vi "PrecessFortran.vi"(0 "Asc reta":string="6.014379870", 1 "Var RA":string="0", 5 "Declinação":string="-0.024612536", 7 "Temperatura (Kelvin)":string="286.45", 9 "Pressao atmosferica (mB)":string="1014", 11 "Humidade relativa (0 a 1)":string=".80", 12 "Var DEC":string="0") -> (3 "Estimated air mass":dbl, 4 "Observed RA (radians)":dbl, 6 "Observed Dec (radians)":dbl, 8 "Observed HA (radians)":dbl, 10 "Local apparent sidereal time (radians)":dbl, 14 "Observed Azimuth (radians: N=0,E=90)":dbl, 15 "Observed Zenith Distance (radians)":dbl)   [LabVIEW 2018]
uses:
  Global_Telescopio.vi
panel:
  in  "Case Constant\n(See Context Help)":bool=TRUE
  out "concatenated string":string
  in  "Taxa de lapso troposferico (Kelvin/metro)":string=".0065"
  in  "Comprimento de onda efetivo (micron)":string=".55"
  in  "Altitude do telescopio":string="1836.4"
  in  "Latitude do telescopio":string="-0.393299281"
  in  "Longitude do telescopio":string="-0.795507013"
  in  "Coord. y do mov. do polo":string="0.000002363"
  in  "Coord. x do mov. do polo":string="0.000000206"
  in  "Delta UT: UT1-UTC":string="-.0776422"
  in  "Data Juliana Modificada":string="54302.384"
  in  "Epoca do equinocio":string="2000"
  in  "Paralaxe":string="0"
  in  "Vel Radial km/seg":string="0"
  out "Arquivo input.txt":string
  out "Arquivo Output.txt":string
  # "Variáveis de entrada"
  # "Variáveis internas"
  # "Constantes"
  # "Variáveis de Saídas"
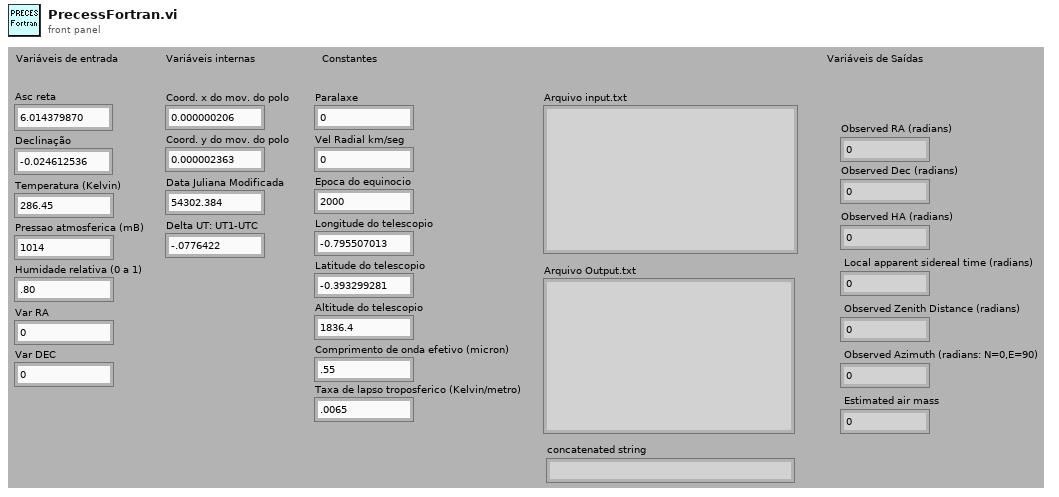
[diagram p1: front panel]
types:
  T1 = enum16{"open", "open or create", "create or replace", "create", "open (read only)"}
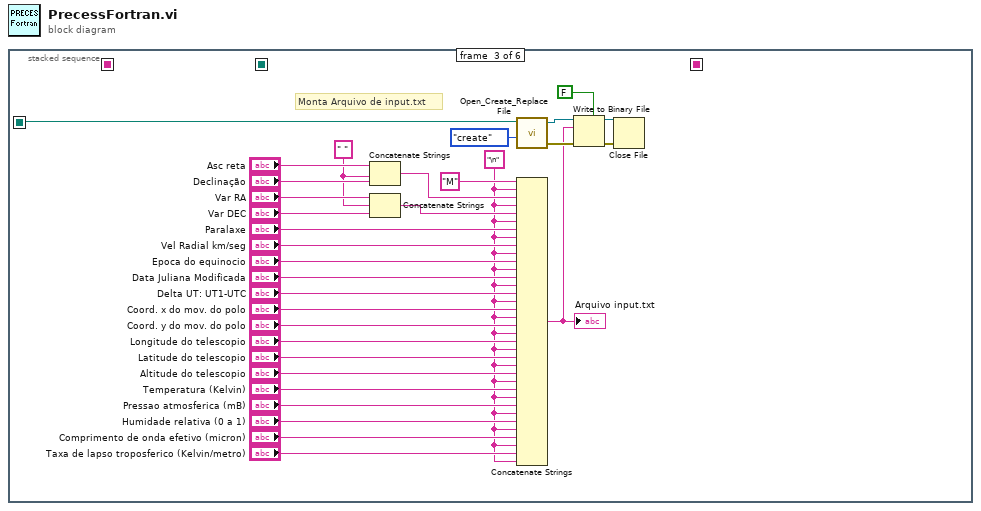
[diagram p0: block diagram]
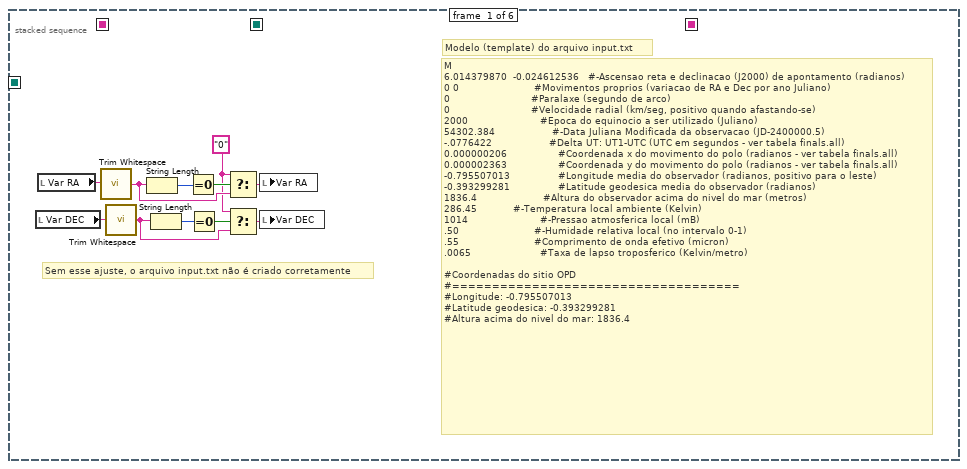
[diagram p2: hidden frame]
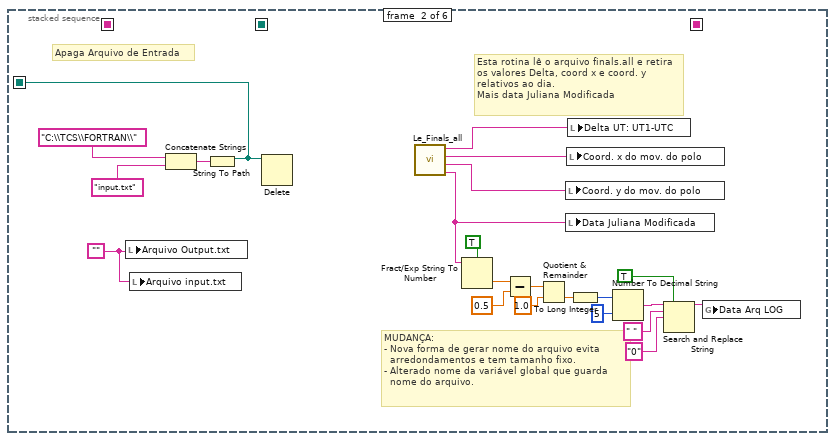
[diagram p3: hidden frame]
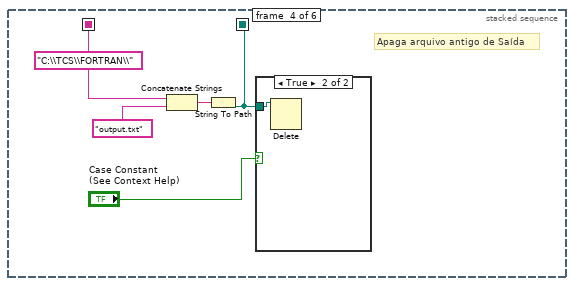
[diagram p4: hidden frame]
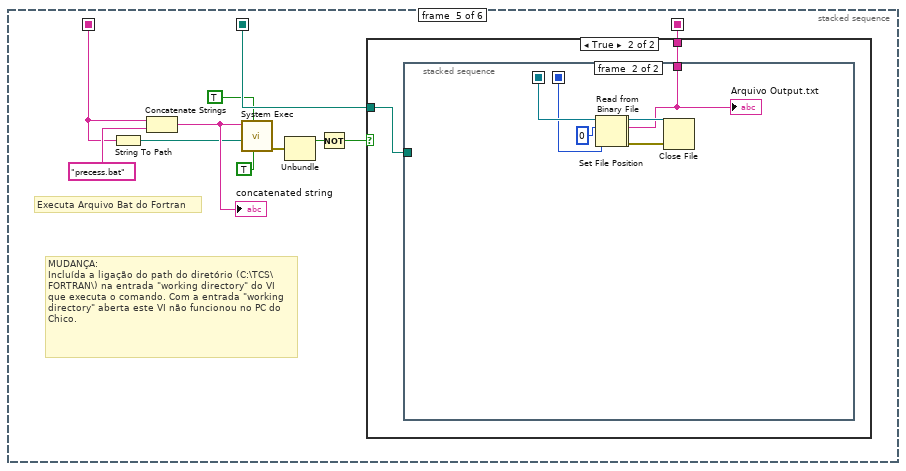
[diagram p6: hidden frame]
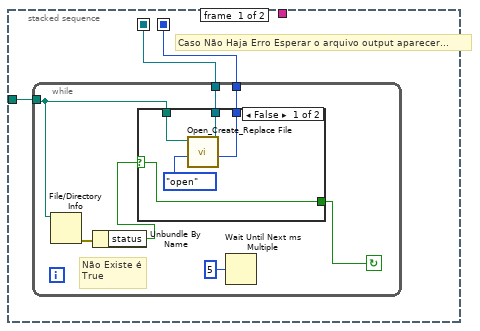
[diagram p8: hidden frame]
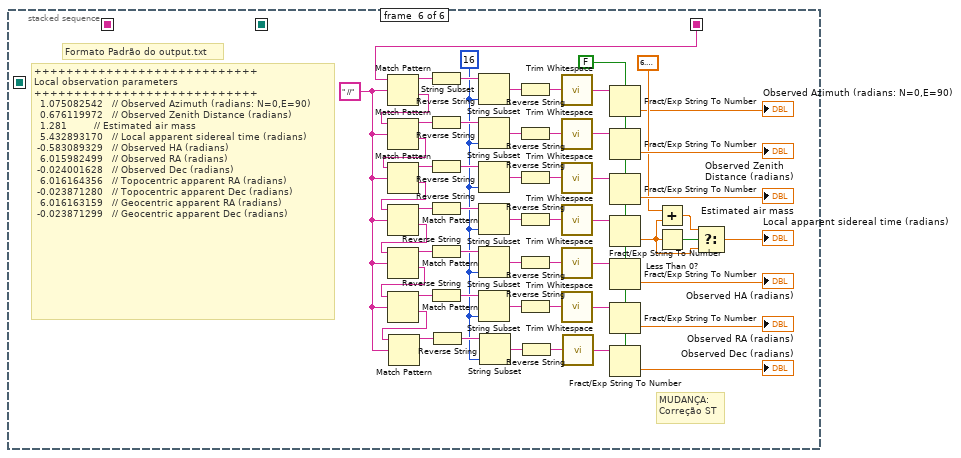
[diagram p10: hidden frame]
diagram:
  n1 = stacked-sequence {
    seq-local: [_ _ _ w70 _ _] -> [_ _ _ _ w72 _]
    seq-local: [_ _ _ w69 _ _] -> [_ _ _ _ w77 _]
    seq-local: [_ w30 _ _ _ _] -> [_ _ w61 _ _ _]
    seq-local: [_ _ _ _ w74 _] -> [_ _ _ _ _ w164]
    frame #0 {
      w3 = "0"
      # "Sem esse ajuste, o arquivo input.txt não é criado corretamente"
      # "Modelo (template) do arquivo input.txt"
      # "M\n6.014379870  -0.024612536   #-Ascensao reta e declinacao (J2000) de apontamento (radianos)\n0 0                         #Movimentos proprios (variacao de RA e Dec por ano Juliano)\n0                           #Paralaxe (segundo de arco)\n0                           #Velocidade radial (km/seg, positivo quando afastando-se)\n2000                        #Epoca do equinocio a ser utilizado (Juliano)\n54302.384                   #-Data Juliana Modificada da observacao (JD-2400000.5)\n-.0776422                   #Delta UT: UT1-UTC (UTC em segundos - ver tabela finals.all)\n0.000000206                 #Coordenada x do movimento do polo (radianos - ver tabela finals.all)\n0.000002363                 #Coordenada y do movimento do polo (radianos - ver tabela finals.all)\n-0.795507013                #Longitude media do observador (radianos, positivo para o leste)\n-0.393299281                #Latitude geodesica media do observador (radianos)\n1836.4                      #Altura do observador acima do nivel do mar (metros)\n286.45      \t\t    #-Temperatura local ambiente (Kelvin)\n1014                        #-Pressao atmosferica local (mB)\n.50                         #-Humidade relativa local (no intervalo 0-1)\n.55                         #Comprimento de onda efetivo (micron)\n.0065                       #Taxa de lapso troposferico (Kelvin/metro)\n\n#Coordenadas do sitio OPD\n#====================================\n#Longitude: -0.795507013\n#Latitude geodesica: -0.393299281\n#Altura acima do nivel do mar: 1836.4"
      n2 = local read "Var DEC"() -> (w10:string)
      n3 = local read "Var RA"() -> (w11:string)
      n4 = call <vilib>:"Trim Whitespace.vi"("string"=w11) -> ("trimmed string"=w5:string)  [unwired: 1 in]
      n5 = call <vilib>:"Trim Whitespace.vi"("string"=w10) -> ("trimmed string"=w4:string)  [unwired: 1 in]
      n6 = String Length(string=w5) -> (length=w9:i32)
      n7 = String Length(string=w4) -> (length=w8:i32)
      n8 = Equal To 0?(x=w9) -> (x = 0?=w7:bool)
      n9 = Equal To 0?(x=w8) -> (x = 0?=w6:bool)
      n10 = Select(t=w3, s=w7, f=w5) -> (s? t:f=w2:string)
      n11 = Select(t=w3, s=w6, f=w4) -> (s? t:f=w1:string)
      n12 = local write "Var RA"(w2) -> ()
      n13 = local write "Var DEC"(w1) -> ()
    }
    frame #1 {
      w29 = ""
      # "MUDANÇA:\n- Nova forma de gerar nome do arquivo evita\n  arredondamentos e tem tamanho fixo.\n- Alterado nome da variável global que guarda\n  nome do arquivo."
      # "Esta rotina lê o arquivo finals.all e retira\nos valores Delta, coord x e coord. y \nrelativos ao dia.\nMais data Juliana Modificada"
      # "Apaga Arquivo de Entrada"
      n14 = local write "Arquivo Output.txt"(w29) -> ()
      n15 = local write "Arquivo input.txt"(w29) -> ()
      n16 = Concatenate Strings("C:\\TCS\\FORTRAN\\", "input.txt") -> (w33:string)
      n17 = String To Path(string=w33) -> (path=w30:path)
      n18 = Delete(path (use dialog)=w30) -> ()  [unwired: 4 in, 3 out]
      n19 = call "Le_Finals_all.vi"() -> ("Data Juliana Modificada"=w25:string, "Saída coord y"=w26:string, "Saída coord x"=w27:string, "Saída DeltaUT"=w28:string)  [unwired: 5 in]
      n20 = Fract/Exp String To Number(use system decimal point (T)=TRUE, string=w25) -> (number=w23:dbl)  [unwired: 2 in, 1 out]
      n21 = Subtract(x=w23, y=0.5) -> (x-y=w13:dbl)
      n22 = Quotient & Remainder(x=w13, y=1.0) -> (floor(x/y)=w15:dbl)  [unwired: 1 out]
      n23 = local write "Coord. y do mov. do polo"(w26) -> ()
      n24 = local write "Data Juliana Modificada"(w25) -> ()
      n25 = local write "Coord. x do mov. do polo"(w27) -> ()
      n26 = local write "Delta UT: UT1-UTC"(w28) -> ()
      n27 = To Long Integer(number=w15) -> (32bit integer=w14:i32)
      n28 = Number To Decimal String(number=w14, width (-)=i16 5) -> (decimal integer string=w20:string)
      n29 = Search and Replace String(replace all?=TRUE ("replace all? (F)"), input string=w20, search string=" ", replace string="0" ("replace string (\"\")")) -> (result string=w12:string)  [unwired: 4 in, 3 out]
      n30 = global write "Global_Telescopio.vi" "Data Arq LOG"(w12) -> ()
    }
    frame #2 {
      w53 = " " ("string")
      w35 = "\n"
      # "Monta Arquivo de input.txt"
      n31 = Concatenate Strings("Asc reta", w53, "Declinação") -> (w57:string)
      n32 = Concatenate Strings("Var RA", w53, "Var DEC") -> (w51:string)
      n33 = call <vilib>:"Open_Create_Replace File.vi"("function (open:0)"=T1."create", "file path"=w61) -> ("error out"=w64:errorcluster, "refnum"=w65:refnum<file>)  [unwired: 6 in, 2 out]
      n34 = Concatenate Strings("M", w35, w57, w35, w51, w35, "Paralaxe", w35, "Vel Radial km/seg", w35, "Epoca do equinocio", w35, "Data Juliana Modificada", w35, "Delta UT: UT1-UTC", w35, "Coord. x do mov. do polo", w35, "Coord. y do mov. do polo", w35, "Longitude do telescopio", w35, "Latitude do telescopio", w35, "Altitude do telescopio", w35, "Temperatura (Kelvin)", w35, "Pressao atmosferica (mB)", w35, "Humidade relativa (0 a 1)", w35, "Comprimento de onda efetivo (micron)", w35, "Taxa de lapso troposferico (Kelvin/metro)", w35) -> (w58:string)
      "Arquivo input.txt" <- w58
      n35 = Write to Binary File(file (use dialog)=w65, data=w58, error in=w64, 5:FALSE ("prepend array or string size? (T)")) -> (refnum out=w62:refnum<file>, error out=w63:errorcluster)  [unwired: 2 in, 1 out]
      n36 = Close File(refnum=w62, error in=w63) -> ()  [unwired: 2 out]
    }
    frame #3 {
      w70 = "C:\\TCS\\FORTRAN\\"
      # "Apaga arquivo antigo de Saída"
      n37 = Concatenate Strings(w70, "output.txt") -> (w68:string)
      n38 = String To Path(string=w68) -> (path=w69:path)
      n39 = case shown="True" "Case Constant\n(See Context Help)" {
        tunnel: w69 -> [_ w71]
        frame False {
        }
        frame True {
          n40 = Delete(path (use dialog)=w71) -> ()  [unwired: 4 in, 3 out]
        }
      }
    }
    frame #4 {
      # "MUDANÇA:\nIncluída a ligação do path do diretório (C:\\TCS\\FORTRAN\\) na entrada \"working directory\" do VI que executa o comando. Com a entrada \"working directory\" aberta este VI não funcionou no PC do Chico."
      # "Executa Arquivo Bat do Fortran"
      n41 = String To Path(string=w72) -> (path=w73:path)
      n42 = Concatenate Strings(w72, "precess.bat") -> (w81:string)
      "concatenated string" <- w81
      n43 = call <vilib>:"System Exec.vi"("run minimized? (F)"=TRUE, "wait until completion? (T)"=TRUE, "working directory"=w73, "command line"=w81) -> ("error out"=w80:errorcluster)  [unwired: 4 in, 3 out]
      n44 = Unbundle(w80) -> ("status"=w79:bool)  [unwired: 2 out]
      n45 = Not(x=w79) -> (.not. x?=w78:bool)
      n46 = case shown="True" w78 {
        tunnel: w77 -> [_ w84]
        tunnel: [_ w83] -> w74
        frame False {
        }
        frame True {
          n47 = stacked-sequence {
            seq-local: [w86 _] -> [_ w108]
            seq-local: [w85 _] -> [_ w104]
            tunnel: w84 -> [w87 _]
            tunnel: [_ w103] -> w83
            frame #0 {
              # "Caso Não Haja Erro Esperar o arquivo output aparecer..."
              n48 = while {
                tunnel: w87 -> [w90]
                tunnel: [w92] -> w86
                tunnel: [w93] -> w85
                stop <- w88 continue-if-true
                # "Não Existe é\nTrue"
                n49 = File/Directory Info(path=w90) -> (error out=w91:errorcluster)  [unwired: 1 in, 6 out]
                n50 = Unbundle By Name(w91) -> ("status"=w89:bool)
                n51 = case shown="False" w89 {
                  selector: w89 -> [w95 w100]
                  tunnel: w90 -> [w99 _]
                  tunnel: [w97 _] -> w93
                  tunnel: [w96 _] -> w92
                  tunnel: [w95 w100] -> w88
                  frame False {
                    n52 = call <vilib>:"Open_Create_Replace File.vi"("function (open:0)"=T1."open", "file path"=w99) -> ("file size (bytes)"=w97:i32, "refnum"=w96:refnum<file>)  [unwired: 6 in, 2 out]
                  }
                  frame True {
                  }
                }
                n53 = Wait Until Next ms Multiple(millisecond multiple=u32 5) -> ()  [unwired: 1 out]
              }
            }
            frame #1 {
              n54 = Set File Position(offset (in bytes) (0)=0 ("pos offset (0)"), refnum=w108) -> (refnum out=w102:refnum<file>, error out=w101:errorcluster)  [unwired: 2 in]
              n55 = Read from Binary File(8:w101, 10:w104, 11:w102) -> (0:w106:errorcluster, 2:w103:string, 3:w107:refnum<file>)  [unwired: 3 in, 1 out]
              "Arquivo Output.txt" <- w103
              n56 = Close File(refnum=w107, error in=w106) -> ()  [unwired: 2 out]
            }
          }
        }
      }
    }
    frame #5 {
      w120 = FALSE ("use system decimal point (T)")
      w129 = 16 ("length (rest)")
      w128 = " //" ("regular expression")
      # "MUDANÇA:\nCorreção ST"
      # "Formato Padrão do output.txt"
      # "++++++++++++++++++++++++++++\nLocal observation parameters\n++++++++++++++++++++++++++++\n  1.075082542   // Observed Azimuth (radians: N=0,E=90) \n  0.676119972   // Observed Zenith Distance (radians) \n  1.281         // Estimated air mass \n  5.432893170   // Local apparent sidereal time (radians) \n -0.583089329   // Observed HA (radians) \n  6.015982499   // Observed RA (radians) \n -0.024001628   // Observed Dec (radians) \n  6.016164356   // Topocentric apparent RA (radians) \n -0.023871280   // Topocentric apparent Dec (radians) \n  6.016163159   // Geocentric apparent RA (radians) \n -0.023871299   // Geocentric apparent Dec (radians)"
      n57 = Match Pattern(string=w164, regular expression=w128) -> (before substring=w163:string, after substring=w151:string)  [unwired: 1 in, 2 out]
      n58 = Match Pattern(string=w151, regular expression=w128) -> (before substring=w156:string, after substring=w150:string)  [unwired: 1 in, 2 out]
      n59 = Match Pattern(string=w150, regular expression=w128) -> (before substring=w155:string, after substring=w133:string)  [unwired: 1 in, 2 out]
      n60 = Match Pattern(string=w133, regular expression=w128) -> (before substring=w149:string, after substring=w132:string)  [unwired: 1 in, 2 out]
      n61 = Match Pattern(string=w132, regular expression=w128) -> (before substring=w145:string, after substring=w131:string)  [unwired: 1 in, 2 out]
      n62 = Match Pattern(string=w131, regular expression=w128) -> (before substring=w141:string, after substring=w130:string)  [unwired: 1 in, 2 out]
      n63 = Match Pattern(string=w130, regular expression=w128) -> (before substring=w134:string)  [unwired: 1 in, 3 out]
      n64 = Reverse String(1:w163) -> (0:w162:string)
      n65 = Reverse String(1:w156) -> (0:w157:string)
      n66 = Reverse String(1:w155) -> (0:w154:string)
      n67 = Reverse String(1:w149) -> (0:w148:string)
      n68 = Reverse String(1:w145) -> (0:w144:string)
      n69 = Reverse String(1:w141) -> (0:w140:string)
      n70 = Reverse String(1:w134) -> (0:w135:string)
      n71 = String Subset(string=w162, length (rest)=w129) -> (substring=w161:string)  [unwired: 1 in]
      n72 = String Subset(string=w157, length (rest)=w129) -> (substring=w158:string)  [unwired: 1 in]
      n73 = String Subset(string=w154, length (rest)=w129) -> (substring=w153:string)  [unwired: 1 in]
      n74 = String Subset(string=w148, length (rest)=w129) -> (substring=w147:string)  [unwired: 1 in]
      n75 = String Subset(string=w144, length (rest)=w129) -> (substring=w143:string)  [unwired: 1 in]
      n76 = String Subset(string=w140, length (rest)=w129) -> (substring=w139:string)  [unwired: 1 in]
      n77 = String Subset(string=w135, length (rest)=w129) -> (substring=w136:string)  [unwired: 1 in]
      n78 = Reverse String(1:w161) -> (0:w160:string)
      n79 = Reverse String(1:w158) -> (0:w159:string)
      n80 = Reverse String(1:w153) -> (0:w152:string)
      n81 = Reverse String(1:w147) -> (0:w146:string)
      n82 = Reverse String(1:w143) -> (0:w142:string)
      n83 = Reverse String(1:w139) -> (0:w138:string)
      n84 = Reverse String(1:w136) -> (0:w137:string)
      n85 = call <vilib>:"Trim Whitespace.vi"("string"=w160) -> ("trimmed string"=w127:string)  [unwired: 1 in]
      n86 = call <vilib>:"Trim Whitespace.vi"("string"=w159) -> ("trimmed string"=w126:string)  [unwired: 1 in]
      n87 = call <vilib>:"Trim Whitespace.vi"("string"=w152) -> ("trimmed string"=w125:string)  [unwired: 1 in]
      n88 = call <vilib>:"Trim Whitespace.vi"("string"=w146) -> ("trimmed string"=w124:string)  [unwired: 1 in]
      n89 = call <vilib>:"Trim Whitespace.vi"("string"=w142) -> ("trimmed string"=w123:string)  [unwired: 1 in]
      n90 = call <vilib>:"Trim Whitespace.vi"("string"=w138) -> ("trimmed string"=w122:string)  [unwired: 1 in]
      n91 = call <vilib>:"Trim Whitespace.vi"("string"=w137) -> ("trimmed string"=w121:string)  [unwired: 1 in]
      n92 = Fract/Exp String To Number(use system decimal point (T)=w120, string=w127) -> (number=→"Observed Azimuth (radians: N=0,E=90)":dbl)  [unwired: 2 in, 1 out]
      n93 = Fract/Exp String To Number(use system decimal point (T)=w120, string=w126) -> (number=→"Observed Zenith Distance (radians)":dbl)  [unwired: 2 in, 1 out]
      n94 = Fract/Exp String To Number(use system decimal point (T)=w120, string=w125) -> (number=→"Estimated air mass":dbl)  [unwired: 2 in, 1 out]
      n95 = Fract/Exp String To Number(use system decimal point (T)=w120, string=w124) -> (number=w112:dbl)  [unwired: 2 in, 1 out]
      n96 = Fract/Exp String To Number(use system decimal point (T)=w120, string=w123) -> (number=→"Observed HA (radians)":dbl)  [unwired: 2 in, 1 out]
      n97 = Fract/Exp String To Number(use system decimal point (T)=w120, string=w122) -> (number=→"Observed RA (radians)":dbl)  [unwired: 2 in, 1 out]
      n98 = Fract/Exp String To Number(use system decimal point (T)=w120, string=w121) -> (number=→"Observed Dec (radians)":dbl)  [unwired: 2 in, 1 out]
      n99 = Add(x=6.283185307179586, y=w112) -> (x+y=w111:dbl)
      n100 = Less Than 0?(x=w112) -> (x < 0?=w114:bool)
      n101 = Select(t=w111, s=w114, f=w112) -> (s? t:f=→"Local apparent sidereal time (radians)":dbl)
    }
  }
